vi "Downsampler.vi"(2 "Input Array":dbl[](array[numeric]) format="%.2f", 3 "Averaging samples":i32=5) -> (0 "Downsampled Array":dbl[](array[numeric]) format="%.2f", 1 "Samples remaining":dbl[](array[numeric]) format="%.2f")   [LabVIEW 2010]
uses:
  <vilib>/Analysis/NI_AALBase.lvlib
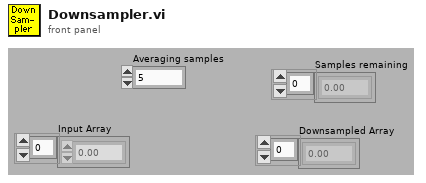
[diagram p1: front panel]
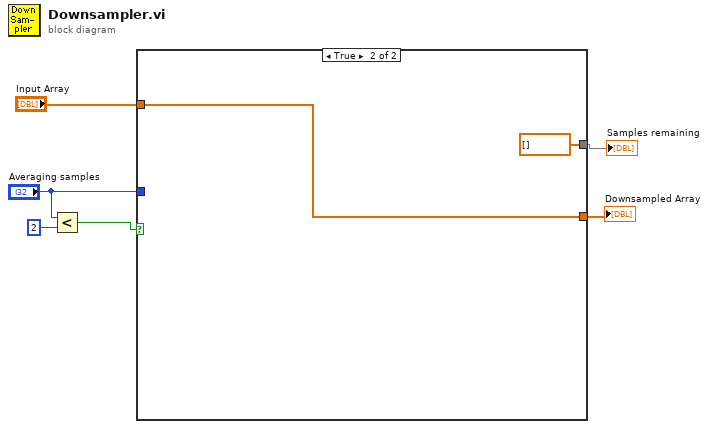
[diagram p0: block diagram]
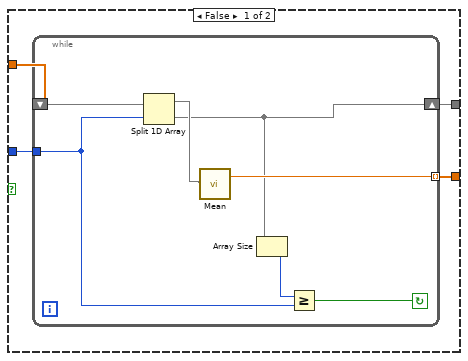
[diagram p2: hidden frame]
diagram:
  n1 = Less?(x="Averaging samples", y=2) -> (x < y?=w1:bool)
  n2 = case shown="True" w1 {
    tunnel: "Input Array" -> [w10 w19]
    tunnel: [w9 w19] -> w5
    tunnel: [w8 dbl[] [] ("Input Array")] -> w4
    tunnel: "Averaging samples" -> [w7 _]
    frame False {
      n3 = while {
        shift-right: [w14] -> w8
        shift-left: w10 -> [w17]
        tunnel: w7 -> [w13]
        tunnel: [w15] -> w9 mode=indexing
        stop <- w12 continue-if-true
        n4 = Split 1D Array(array=w17, index=w13) -> (first subarray=w16:dbl[], second subarray=w14:dbl[])
        n5 = call <vilib>:"Mean.vi"("X"=w16) -> ("mean"=w15:dbl)  [unwired: 1 out]
        n6 = Array Size(array=w14) -> (size(s)=w11:i32)
        n7 = Greater Or Equal?(x=w11, y=w13) -> (x >= y?=w12:bool)
      }
    }
    frame True {
    }
  }
  "Downsampled Array" <- w5
  "Samples remaining" <- w4
